vi "agilent_to_FC.vi"(9 "force curve":dbl[][](array[numeric]), 10 "deflection sensitivity ref":refnum<vi>, 11 "Force constant ref":refnum<vi>) -> (3 "force curve":dbl[][](array[numeric]))   [LabVIEW 2015]
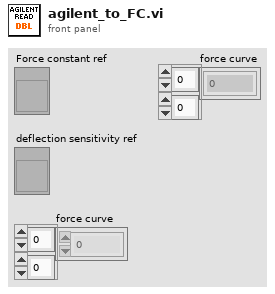
[diagram p1: front panel]
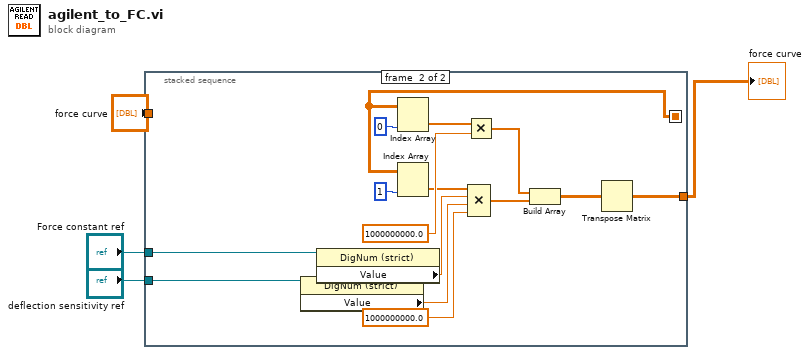
[diagram p0: block diagram]
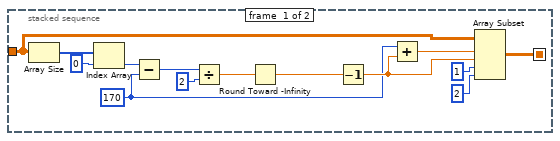
[diagram p2: hidden frame]
diagram:
  n1 = stacked-sequence {
    seq-local: [w17 _] -> [_ w31]
    tunnel: "force curve" -> [w16 _]
    tunnel: [_ w25] -> w4
    tunnel: "Force constant ref" -> [_ w20]
    tunnel: "deflection sensitivity ref" -> [_ w19]
    frame #0 {
      w5 = 170 ("index")
      n2 = Array Size(array=w16) -> (size(s)=w15:i32[])
      n3 = Index Array(array=w15, index=0) -> (element=w7:i32)
      n4 = Subtract(x=w7, y=w5) -> (x-y=w6:i32)
      n5 = Divide(x=w6, y=2) -> (x/y=w11:dbl)
      n6 = Round Toward -Infinity(1:w11) -> (0:w12:dbl)
      n7 = Decrement(x=w12) -> (x-1=w8:dbl)
      n8 = Add(x=w5, y=w8) -> (x+y=w10:dbl)
      n9 = Array Subset(array=w16, index (row)=w10, length (row)=w8, index (col)=1 ("index"), length (col)=2 ("index")) -> (w17:dbl[][])
    }
    frame #1 {
      n10 = property class="DigNum (strict)"(reference=w19) -> ("Value"=w29:dbl)  [unwired: 1 in, 2 out]
      n11 = property class="DigNum (strict)"(reference=w20) -> ("Value"=w30:dbl)  [unwired: 1 in, 2 out]
      n12 = Index Array(array=w31, index (col)=0 ("disabled index (col)")) -> (element=w21:dbl[])  [unwired: 1 in]
      n13 = Index Array(array=w31, index (col)=1 ("disabled index (col)")) -> (element=w24:dbl[])  [unwired: 1 in]
      n14 = Multiply(x=w21, y=1000000000.0) -> (x*y=w22:dbl[])
      n15 = Compound Arithmetic op=MULTIPLY(w24, w30, w29, 1000000000.0) -> (w23:dbl[])
      n16 = Build Array(w22, w23) -> (w26:dbl[][])
      n17 = Transpose Matrix(1:w26) -> (0:w25:dbl[][])
    }
  }
  "force curve" <- w4
